vi "NOSAMSBouncerDAQrestartFC.vi"(8 "error in (no error)":errorcluster) -> (0 "error out":errorcluster, 2 "Summary Data":T3={"C12LE"=1.472651644671806e-07, "C13LE"=7.43208703350402e-08, "C12"=7.325707563373238e-08, "C13L"=240.0, "C13H"=6.302996266666667, "C1312"=6.305409493333333, "Counts"=0, "LT"=1.0021241544060013, "RT"=0.0, "BadBlocks"=0}, 3 "Run Average Ratios":T7={"C14Rate"=38.07712869341802, "CountErr"=0.06454972243679029, "DT"=0.002413226666666546, "DTfrac"=0.0003827232266545153, "C13"=307109705561.01575, "C13H/L"=0.9856864606602128, "d13C"=-48.24793286826845, "C14/13"=1.23985429323571e-10, "C12Cor"=28715190239906.207, "C13/12"=0.010695028328772694, "C14/12"=1.3260273874313845e-12, "LEC13/12"=0.0} {"LEC13/12" format="%_4e"; "DTfrac" format="%#_3g"; "DT" format="%#_3g"; "CountErr" format="%#_3g"; "d13C" format="%_4g"; "C13/12" format="%_4e"; "C14/12" format="%_4e"; "C14/13" format="%_3e"; "C12Cor" format="%_3e"; "C13" format="%_3e"; "C13H/L" format="%#_3g"})   [LabVIEW 2013]
uses:
  PixieKeithleyDAQstates.ctl
  <vilib>/DAQmx/configure/timing.llb/DAQmx Timing (Sample Clock).vi
  <vilib>/DAQmx/create/channels.llb/DAQmx Create Channel (AI-Voltage-Basic).vi
  <vilib>/DAQmx/create/channels.llb/DAQmx Create Channel (CI-Count Edges).vi
  <vilib>/DAQmx/read.llb/DAQmx Read (Counter U32 1Chan 1Samp).vi
  <vilib>/DAQmx/create/channels.llb/DAQmx Create Channel (CO-Pulse Generation-Time).vi
  <vilib>/DAQmx/configure/timing.llb/DAQmx Timing (Implicit).vi
  <vilib>/DAQmx/create/channels.llb/DAQmx Create Channel (AO-Voltage-Basic).vi
  <vilib>/DAQmx/configure/timing.llb/DAQmx Timing (Use Waveform).vi
  <vilib>/DAQmx/write.llb/DAQmx Write (Analog Wfm 1Chan NSamp).vi
  <resource>/objmgr/daqmx.rc
  <vilib>/DAQmx/configure/trigger.llb/DAQmx Start Trigger (Digital Edge).vi
  <vilib>/DAQmx/read.llb/DAQmx Read (Analog 1D Wfm NChan NSamp).vi
  RunRatios.ctl
  FCOffset.ctl
  SummaryData.ctl
  BouncerParameters.ctl
panel:
  out "Bouncer Waveform":waveform(dbl)(graph)
  in  "Bouncer Parameters":T1={"12C Period"=1.0, "12C Delay"=0.0, "12C Voltage"=9.022, "13C Period"=10.0, "13C Delay"=0.0, "13C Voltage"=5.239, "14C Period"=100.0, "14C Delay"=0.0, "14C Voltage"=2.0, "LE13C Period"=0.0, "LE13C Delay"=0.0, "LE13C Voltage"=0.0, "LE12C Period"=0.0, "LE12C Delay"=0.0, "LE12C Voltage"=0.0} {"LE12C Voltage" format="%_4f"; "LE13C Voltage" format="%_4f"}
  in  "samples per channel":i32=1000
  out "CH1 GDT":dbl
  out "CH0 GDT":dbl
  in  "FC Offset":T2={"HE 12C Offset"=0.0, "HE 13CL Offset"=0.0, "HE 13CH Offset"=0.0, "LE FC Scale"=0, "HE C12 Scale"=0, "HE C13 Scale"=18} {"HE C13 Scale" items=["500 mA/V", "200 mA/V", "100 mA/V", "50 mA/V", "20 mA/V", "10 mA/V", "5 mA/V", "2 mA/V", "1 mA/V", "500 uA/V", "200 uA/V", "100 uA/V", "50 uA/V", "20 uA/V", "10 uA/V", "5 uA/V", "2 uA/V", "1 uA/V", "500 nA/V", "200 nA/V", "100 nA/V", "50 nA/V", "20 nA/V", "10 nA/V", "5 nA/V", "2 nA/V", "1 nA/V", "500 pA/V", "200 pA/V", "100 pA/V", "50 pA/V", "20 pA/V", "10 pA/V", "5 pA/V", "2 pA/V", "1 pA/V", ""]; "HE C12 Scale" items=["500 mA/V", "200 mA/V", "100 mA/V", "50 mA/V", "20 mA/V", "10 mA/V", "5 mA/V", "2 mA/V", "1 mA/V", "500 uA/V", "200 uA/V", "100 uA/V", "50 uA/V", "20 uA/V", "10 uA/V", "5 uA/V", "2 uA/V", "1 uA/V", "500 nA/V", "200 nA/V", "100 nA/V", "50 nA/V", "20 nA/V", "10 nA/V", "5 nA/V", "2 nA/V", "1 nA/V", "500 pA/V", "200 pA/V", "100 pA/V", "50 pA/V", "20 pA/V", "10 pA/V", "5 pA/V", "2 pA/V", "1 pA/V", ""]; "LE FC Scale" items=["500 mA/V", "200 mA/V", "100 mA/V", "50 mA/V", "20 mA/V", "10 mA/V", "5 mA/V", "2 mA/V", "1 mA/V", "500 uA/V", "200 uA/V", "100 uA/V", "50 uA/V", "20 uA/V", "10 uA/V", "5 uA/V", "2 uA/V", "1 uA/V", "500 nA/V", "200 nA/V", "100 nA/V", "50 nA/V", "20 nA/V", "10 nA/V", "5 nA/V", "2 nA/V", "1 nA/V", "500 pA/V", "200 pA/V", "100 pA/V", "50 pA/V", "20 pA/V", "10 pA/V", "5 pA/V", "2 pA/V", "1 pA/V", ""]}
  out "HE 13CL Cup":waveform(dbl)(graph)={"t0"=timestamp(3415120333.4017754 s since 1904-01-01), "dt"=9.999999999999972e-06, "Y"=[0.41889009921070675, 0.6410939957678486, 0.7270772818431984, 0.7261111773784867, 0.7270772818431984, 0.7293315256055366, 0.7267552470213039, 0.7286874559575331, 0.7306196649054364, 0.7254671077369653, 0.7283654211340178, 0.7302976300799747, 0.7277213514879598, 0.7261111773784867, 0.7306196649054364, 0.7341620480069433, 0.7293315256055366, 0.7302976300799747, 0.7319078042105287, 0.7331959435208164, 0.7280433863108267, 0.7331959435208164, 0.7290094907813727, 0.7299755952548376, 0.7309416997312226, 0.7344840828363023, 0.7293315256055366, 0.7299755952548376, 0.7267552470213039, 0.7338400131779094, 0.7219247247317432, 0.7225687943661443, 0.7280433863108267, 0.7280433863108267, 0.7309416997312226, 0.7290094907813727, 0.7328739086927573, 0.7277213514879598, 0.7161280980802982, 0.7286874559575331], "attributes"=variant("NI_ChannelName"=variant(string "PXI1Slot2/ai2"), "NI_UnitDescription"=variant(string "Volts"))}
  out "Bouncer":waveform(dbl)(graph)={"t0"=timestamp(3415120333.4009705 s since 1904-01-01), "dt"=9.999999999999972e-06, "Y"=array[1000 elements], "attributes"=variant("NI_ChannelName"=variant(string "PXI1Slot2/ai0"), "NI_UnitDescription"=variant(string "Volts"))}
  out "LE 13C Cup":waveform(dbl)(graph)={"t0"=timestamp(3415120333.402178 s since 1904-01-01), "dt"=9.999999999999972e-06, "Y"=[0.8050097183722652, 0.24660166407635983, 0.028584441505206795, 0.009584422869030943, 0.009906457076575987, 0.00797425183471986, 0.00797425183471986, 0.007008149216862962, 0.012804764954733521, 0.01312679916455761, 0.010550525492349248, 0.010872559700577551, 0.009584422869030943, 0.01022849128434874, 0.01151662811771772, 0.010872559700577551, 0.010872559700577551, 0.010872559700577551, 0.01022849128434874, 0.009262388661713566, 0.004109841375562904, 0.009262388661713566, 0.01151662811771772, 0.01022849128434874, 0.019567483409006912, 0.01151662811771772, 0.010872559700577551, 0.009906457076575987, 0.009584422869030943, 0.01022849128434874, 0.013448833374609843, 0.01022849128434874, 0.009906457076575987, 0.010550525492349248, 0.00668611501136536, 0.010550525492349248, 0.01022849128434874, 0.01022849128434874, 0.009584422869030943, 0.013448833374609843], "attributes"=variant("NI_ChannelName"=variant(string "PXI1Slot2/ai3"), "NI_UnitDescription"=variant(string "Volts"))}
  out "LE 12C Cup":waveform(dbl)(graph)={"t0"=timestamp(3415120333.4013777 s since 1904-01-01), "dt"=9.999999999999972e-06, "Y"=[0.00668611501136536, 0.007008149216862962, 0.007652217628540168, 0.007330183422587883, 0.00861832024776164, 0.007330183422587883, 0.009262388661713566, 0.01312679916455761, 0.05338107720327494, 0.6781279926088322, 0.8175690797952145, 0.8223996035554544, 0.8240097781590372, 0.8233657083165931, 0.8249758829252316, 0.8230436733958766, 0.8243318130807649, 0.8236877432376466, 0.8243318130807649, 0.8243318130807649, 0.8233657083165931, 0.8278741972420289, 0.8236877432376466, 0.8240097781590372, 0.8227216384754971, 0.8246538480028296, 0.8246538480028296, 0.8246538480028296, 0.8249758829252316, 0.8252979178479707, 0.8214334987973474, 0.8236877432376466, 0.8246538480028296, 0.8246538480028296, 0.8227216384754971, 0.8236877432376466, 0.8243318130807649, 0.8217555337163797, 0.8240097781590372, 0.8243318130807649], "attributes"=variant("NI_ChannelName"=variant(string "PXI1Slot2/ai3"), "NI_UnitDescription"=variant(string "Volts"))}
  out "HE 13CH Cup":waveform(dbl)(graph)={"t0"=timestamp(3415120333.4017754 s since 1904-01-01), "dt"=9.999999999999972e-06, "Y"=[0.41889009921070675, 0.6410939957678486, 0.7270772818431984, 0.7261111773784867, 0.7270772818431984, 0.7293315256055366, 0.7267552470213039, 0.7286874559575331, 0.7306196649054364, 0.7254671077369653, 0.7283654211340178, 0.7302976300799747, 0.7277213514879598, 0.7261111773784867, 0.7306196649054364, 0.7341620480069433, 0.7293315256055366, 0.7302976300799747, 0.7319078042105287, 0.7331959435208164, 0.7280433863108267, 0.7331959435208164, 0.7290094907813727, 0.7299755952548376, 0.7309416997312226, 0.7344840828363023, 0.7293315256055366, 0.7299755952548376, 0.7267552470213039, 0.7338400131779094, 0.7219247247317432, 0.7225687943661443, 0.7280433863108267, 0.7280433863108267, 0.7309416997312226, 0.7290094907813727, 0.7328739086927573, 0.7277213514879598, 0.7161280980802982, 0.7286874559575331], "attributes"=variant("NI_ChannelName"=variant(string "PXI1Slot2/ai2"), "NI_UnitDescription"=variant(string "Volts"))}
  out "HE 12C Cup":waveform(dbl)(graph)={"t0"=timestamp(3415120333.400973 s since 1904-01-01), "dt"=9.999999999999972e-06, "Y"=[-0.00168677425192447, 0.003143738765882537, -0.002652876849375083, -0.00168677425192447, 0.0008894993512310448, -0.002652876849375083, 0.0005674651500443148, -0.000720671652438485, 0.0018556019561503992, 0.0018556019561503992, 0.0024996703605630385, 0.0015335677542840436, 0.002177636158243383, -0.0013647400523220184, 0.005397978191647298, 0.0018556019561503992, 0.0012115335526442733, 0.0015335677542840436, 0.016669175487689536, 0.2607711773435167, 0.6375516136789285, 0.6369075442122739, 0.6423821347186465, 0.6456024821175347, 0.6449584126352536, 0.6423821347186465, 0.6456024821175347, 0.6427041694571275, 0.639805856822051, 0.6427041694571275, 0.6388397526159826, 0.6449584126352536, 0.6423821347186465, 0.6443143431542244, 0.6452804473762376, 0.6401278915580318, 0.6410939957678486, 0.6468906210858548, 0.6446363778945825, 0.6433482389350278], "attributes"=variant("NI_ChannelName"=variant(string "PXI1Slot2/ai1"), "NI_UnitDescription"=variant(string "Volts"))}
  out "C13LE":dbl=7.360825676338929e-08 format="%_4g"
  out "C12LE":dbl=7.360825676338929e-08 format="%_4g"
  in  "SampClk.Rate":dbl=10000.0
  out "DT Corrected Rate":dbl=38.103932081925684
  out "SCA Rate":dbl=38.473667612740456
  out "SCA Counts":u32=244
  out "CH1 SFDT":dbl=0.004433706666666666 format="%#_2f"
  out "CH0 SFDT":dbl=0.004324053333333333 format="%#_2f"
  in  "Mode":enum16{"Tuning", "Run", "Manual"}(ring)
  out "Block Spectrum":u32[][](graph) caption="ADC Spectrum"
  out "RunningAverages":T3={"C12LE"=1.4726514132603862e-07, "C13LE"=7.431122697335651e-08, "C12"=7.326197420828519e-08, "C13L"=222.0, "C13H"=5.887767893333334, "C1312"=5.884231466666667, "Counts"=0, "LT"=1.0020921000294485, "RT"=0.0, "BadBlocks"=0}
  out "Elapsed Time":dbl=6.3420000000000005
  out "element":T4=enum."Idle"
  in  "Stop":bool
  in  "Stop DAQ":bool
  in  "Run Parameters":T5={"Block time (s)"=0.2, "Max Runtime (s)"=100000.0, "Max Counts"=100000, "C12 Limit"=-1.0, "Max BadBlocks"=100} {"Block time (s)" min=0.0 max=100.0 step=0.1}
  out "Acquiring":bool
  in  "StartDAQ":bool
  in  "Logfile":string="Feb12.txt"
  in  "Log File Path":path=path "C:/DAQ Logs"
  out "Good Block":bool=TRUE
  out "Currents & Counts":cluster{dbl, dbl, dbl, dbl, dbl}(graph)
  out "Ratios":T6(graph)={"C14/12"=1.3260273874313845e-12, "C14/12"=1.3130784198635677e-12, "d13C"=-48.24793286826845, "d13C"=-48.27837602145524}
  out "13C H/L":dbl(knob)=0.9886607752123965 scale=0.0..2.0 scale format="%#_3g"
  out "Currents":cluster{dbl, dbl}(knob)={1.4754487124301994e-07, 1.4806074705013686e-07} scale=0.0..1e-06 scale format="%#_1e"
  out "12/13":dbl=93.50437948492602
  out "Ch1 Rate 2":cluster{dbl, "Ch1 Rate":dbl}(graph)={38.07712869341802, "Ch1 Rate"=37.7052907013146}
  out "Moving Averages":T7={"C14Rate"=37.7052907013146, "CountErr"=0.06711560552140243, "DT"=-0.0035364266666668698, "DTfrac"=-0.0006010006041910865, "C13"=307099831658.9964, "C13H/L"=0.9858802928197172, "d13C"=-48.27837602145524, "C14/13"=1.2277861077821284e-10, "C12Cor"=28715185727621.875, "C13/12"=0.010694686232971703, "C14/12"=1.3130784198635677e-12, "LEC13/12"=0.0} {"LEC13/12" format="%_4e"; "DTfrac" format="%#_3g"; "DT" format="%#_3g"; "CountErr" format="%#_3g"; "d13C" format="%_4g"; "C13/12" format="%_4e"; "C14/12" format="%_4e"; "C14/13" format="%_3e"; "C12Cor" format="%_3e"; "C13" format="%_3e"; "C13H/L" format="%#_3g"}
  in  "CountPoints":i32=30 min=1
  in  "CurPoints":i32=30 min=1
  out "C12":dbl=1.4754487124301994e-07 format="%_4g"
  out "C13L":dbl=7.445249028674759e-08 format="%_4g"
  out "C13H":dbl=7.360825676338929e-08 format="%_4g"
  out "Run time [s]":dbl=6.305409493333333 format="%_6g"
  out "Ch1 LT":dbl=6.302996266666667
  out "Ch1 Counts":u32=240
  out "Ch1 Rate":dbl=38.07712869341802
  out "Ch0 LT":dbl=6.305354879999999
  out "Ch0 Counts":u32=243
  out "Ch0 Rate":dbl=38.53867143477895
  # "Currents"
  # "Counts"
  # "Livetime"
  # "Rate"
  # "SFDT"
  # "GDT"
  # "Cor Rate"
  # "Ch 0"
  # "Ch1"
  # "SCA"
  # "ms"
  # "us"
  # "kV"
  # "ms"
  # "us"
  # "kV"
  # "ms"
  # "us"
  # "kV"
  # "ms"
  # "us"
  # "kV"
  # "ms"
  # "us"
  # "kV"
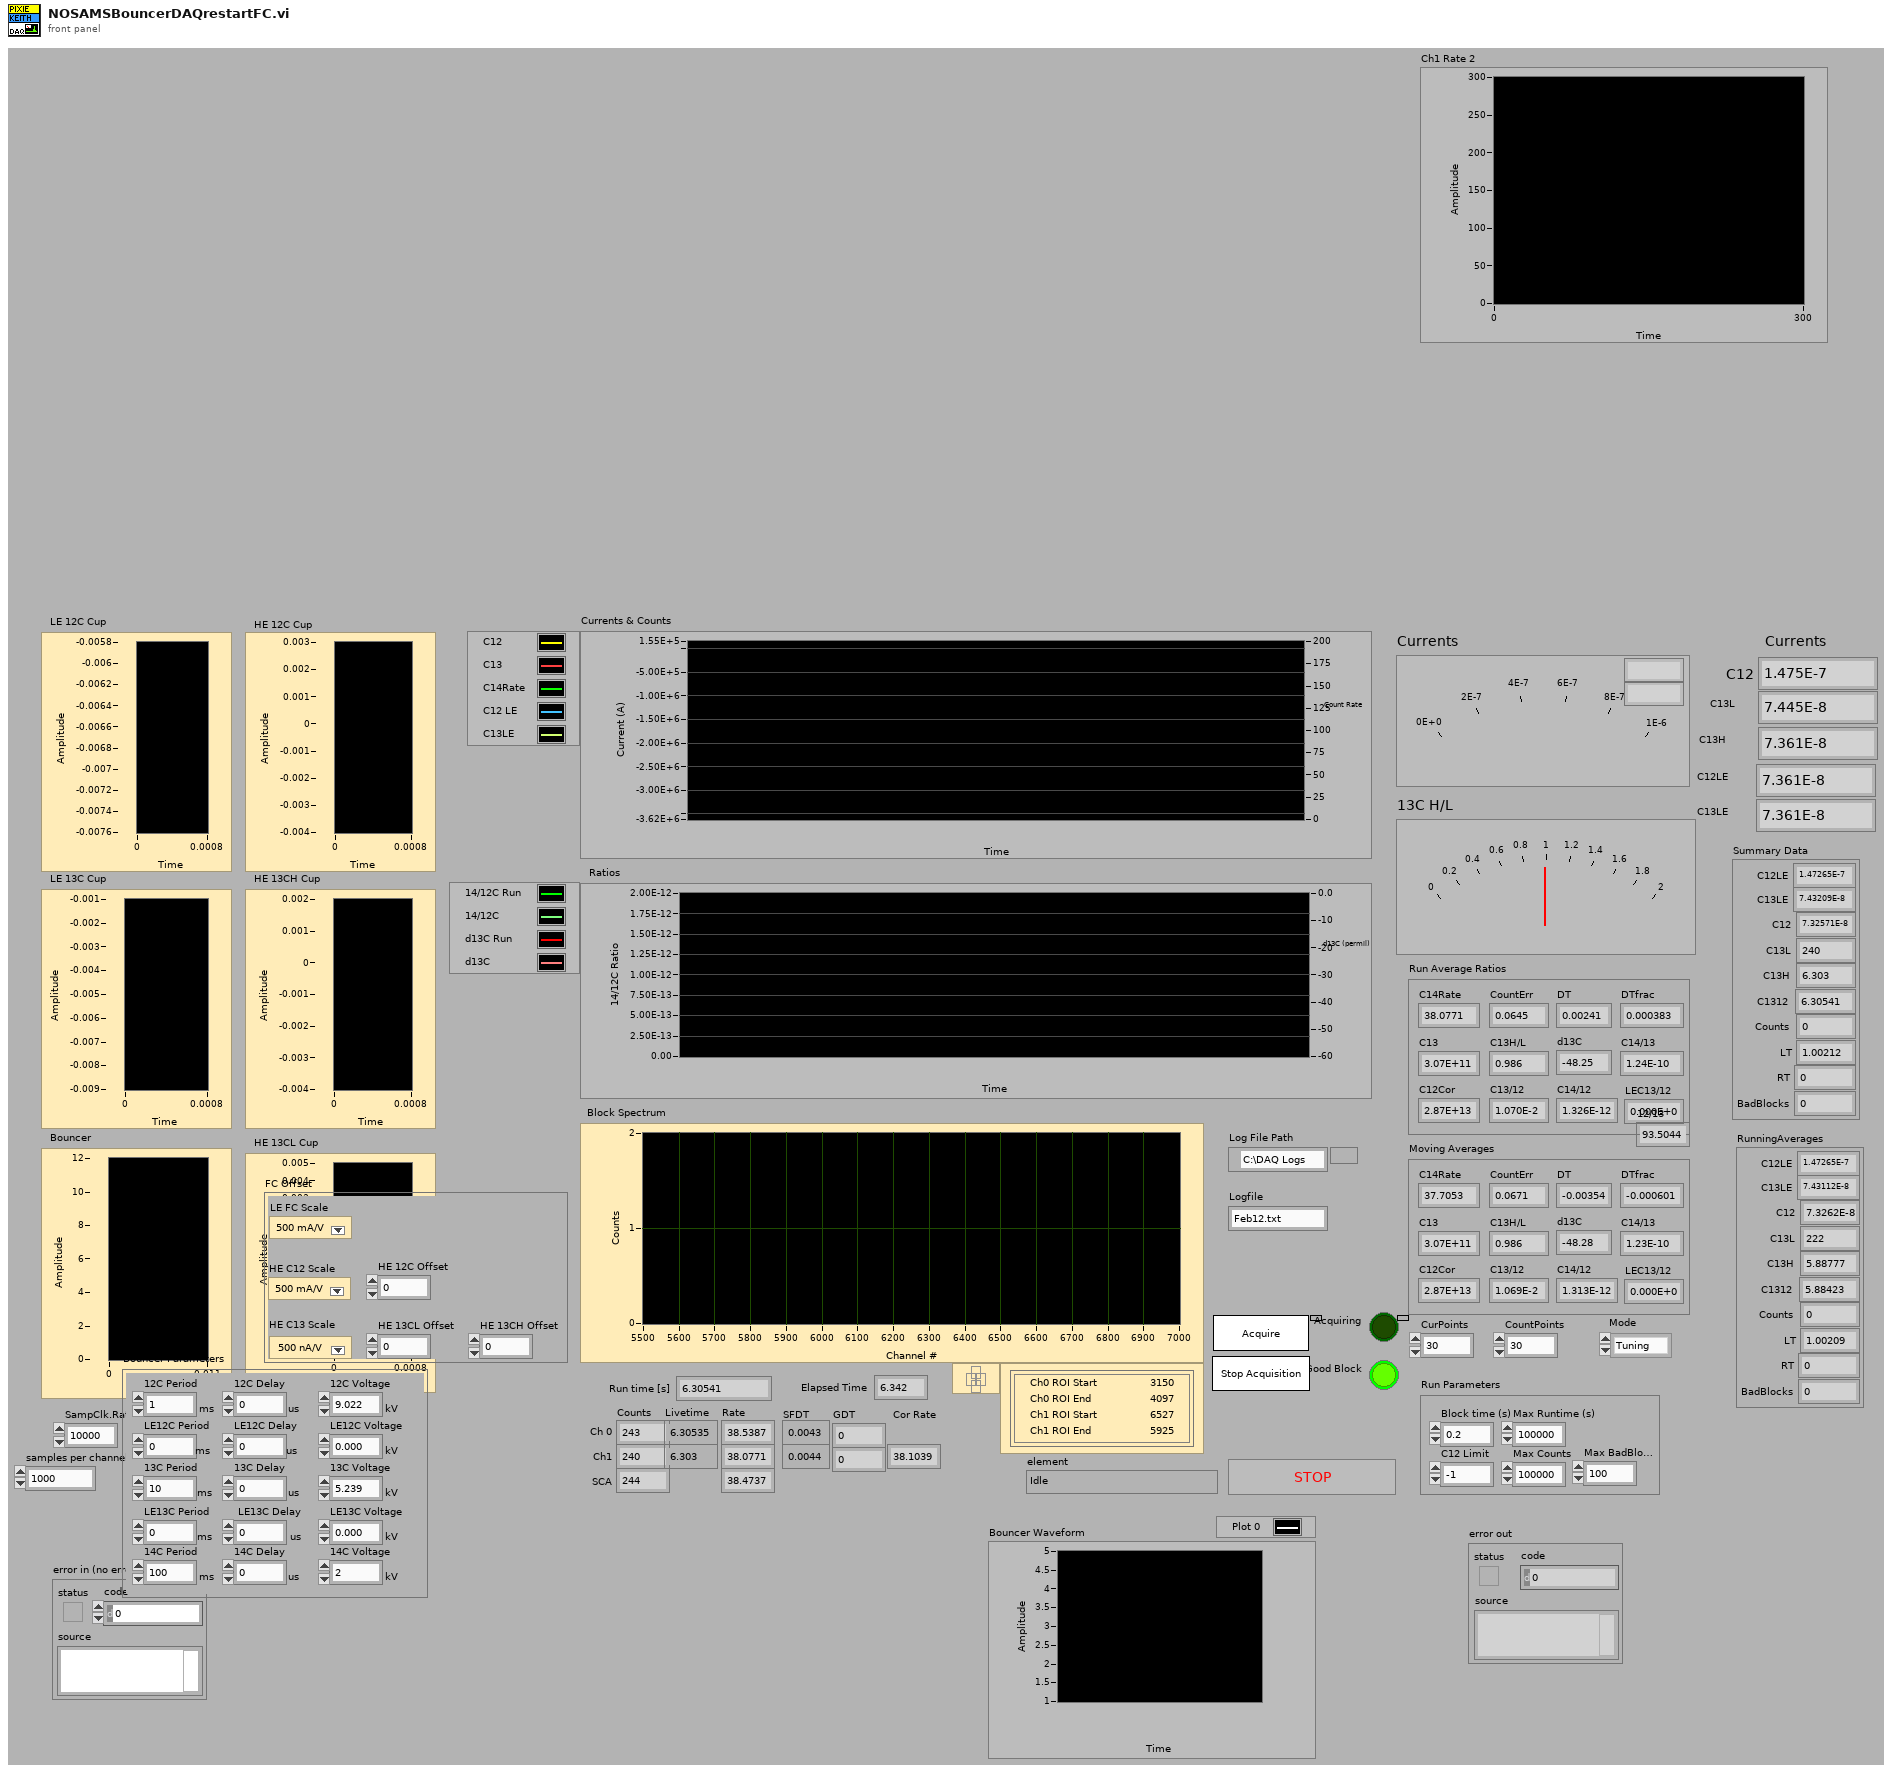
[diagram p1: front panel]
types:
  T1 = typedef "BouncerParameters.ctl" = cluster{"12C Period":dbl, "12C Delay":dbl, "12C Voltage":dbl, "13C Period":dbl, "13C Delay":dbl, "13C Voltage":dbl, "14C Period":dbl, "14C Delay":dbl, "14C Voltage":dbl, "LE13C Period":dbl, "LE13C Delay":dbl, "LE13C Voltage":dbl, "LE12C Period":dbl, "LE12C Delay":dbl, "LE12C Voltage":dbl}
  T2 = typedef "FCOffset.ctl" = cluster{"HE 12C Offset":dbl, "HE 13CL Offset":dbl, "HE 13CH Offset":dbl, "LE FC Scale":u16, "HE C12 Scale":u16, "HE C13 Scale":u16}
  T3 = typedef "SummaryData.ctl" = cluster{"C12LE":dbl, "C13LE":dbl, "C12":dbl, "C13L":dbl, "C13H":dbl, "C1312":dbl, "Counts":u32, "LT":dbl, "RT":dbl, "BadBlocks":u8}
  T4 = typedef "PixieKeithleyDAQstates.ctl" = enum16{"Initialize", "Restart Bouncer", "Idle", "Load Wheel", "Load Sample", "Start Run", "Wait", "Get Block", "Check Data", "Check Run", "Check Sample", "Analyse and Display", "Stop DAQ", "Log Data", "Stop"}
  T5 = cluster{"Block time (s)":dbl, "Max Runtime (s)":dbl, "Max Counts":u32, "C12 Limit":dbl, "Max BadBlocks":u8}
  T6 = cluster{"C14/12":dbl, "C14/12":dbl, "d13C":dbl, "d13C":dbl}
  T7 = typedef "RunRatios.ctl" = cluster{"C14Rate":dbl, "CountErr":dbl, "DT":dbl, "DTfrac":dbl, "C13":dbl, "C13H/L":dbl, "d13C":dbl, "C14/13":dbl, "C12Cor":dbl, "C13/12":dbl, "C14/12":dbl, "LEC13/12":dbl}
  T8 = typedef "BlockData.ctl" = cluster{"LE C12":dbl[], "LE C13":dbl[], "C12":dbl[], "C13L":dbl[], "C13H":dbl[], "C1312":dbl[], "Counts":u32[], "LT":dbl[], "RT":dbl[]}
  T9 = typedef "PixieTimes.ctl" = cluster{"CH0 LT":dbl, "CH1 LT":dbl, "CH0 SFDT":dbl, "CH1 SFDT":dbl, "CH0 GDT":dbl, "CH1 GDT":dbl, "Run time [s]":dbl}
  T10 = typedef "LVCursorListTypeDef.ctl" = cluster{"Name":string, "Color":u32, "Style":u8, "Point Style":u8, "Name Visible":bool, "Allow Drag":bool, "Cursor Mode":u32, "Plot":i32, "Index":i32, "Position":cluster{"X":dbl, "Y":dbl}, "X Scale":u32, "Y Scale":u32, "Watch Plots":i32[], "Watch All Plots":bool, "Plot Area":i32, "Label Offset":cluster{"X":dbl, "Y":dbl}}[]
  T11 = cluster{"Ch0 Counts":u32, "Ch0 Rate":dbl, "Ch1 Counts":u32, "Ch1 Rate":dbl}
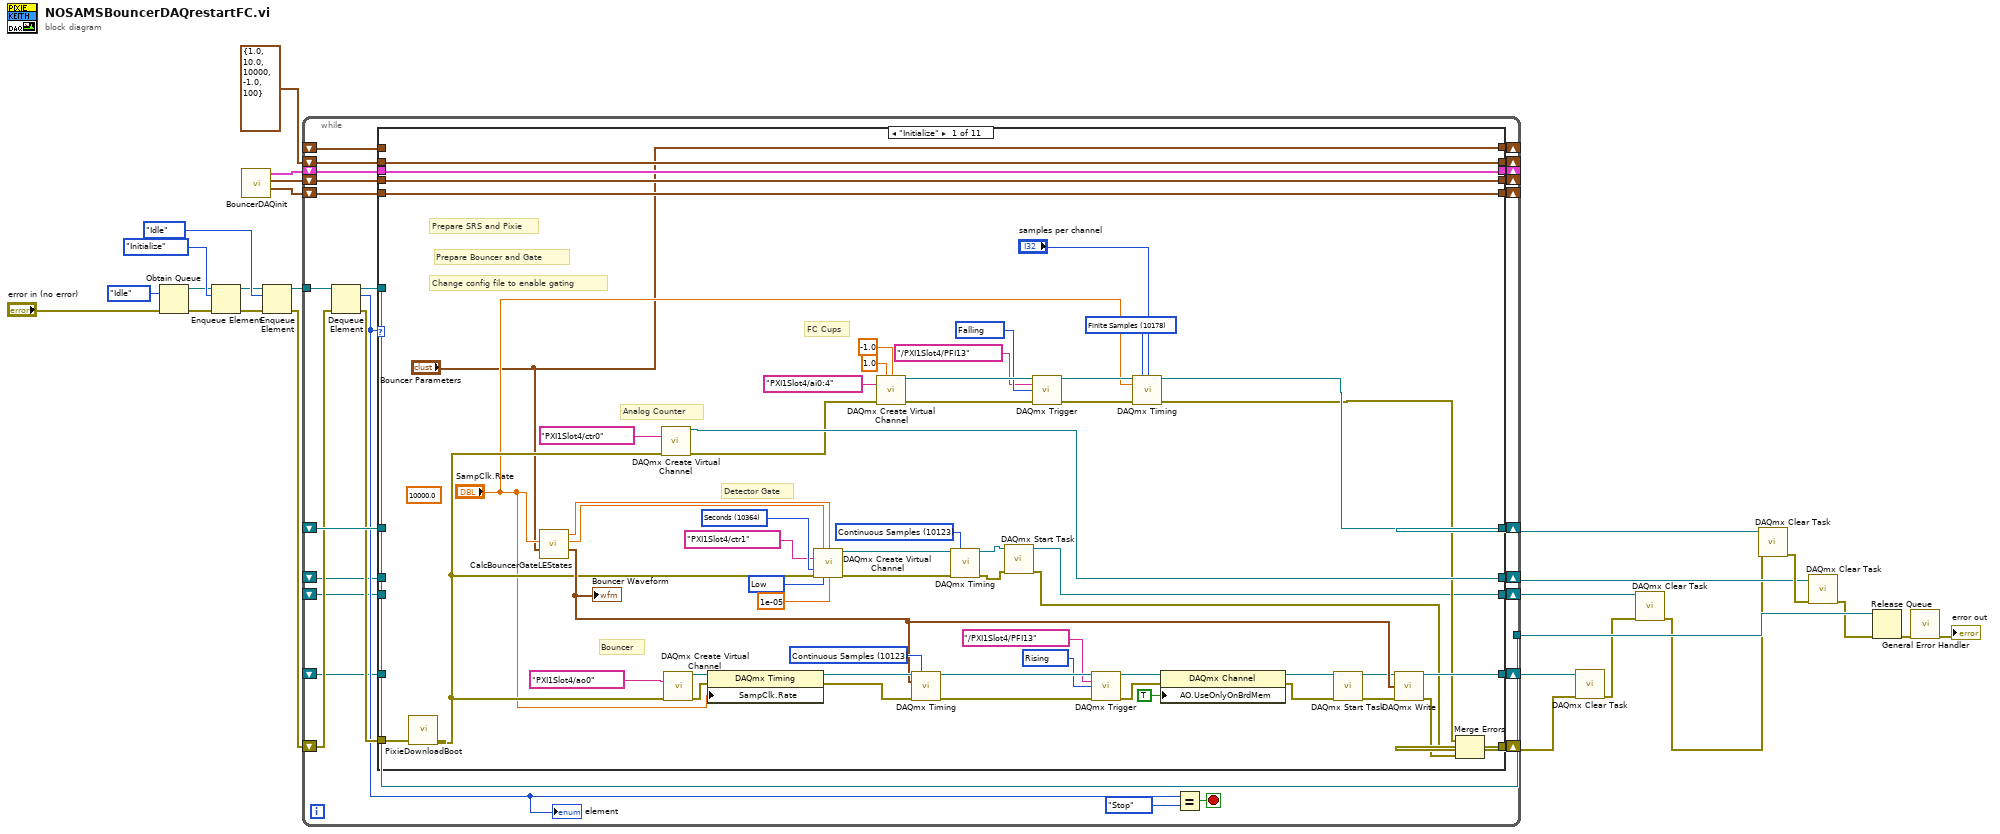
[diagram p0: block diagram]
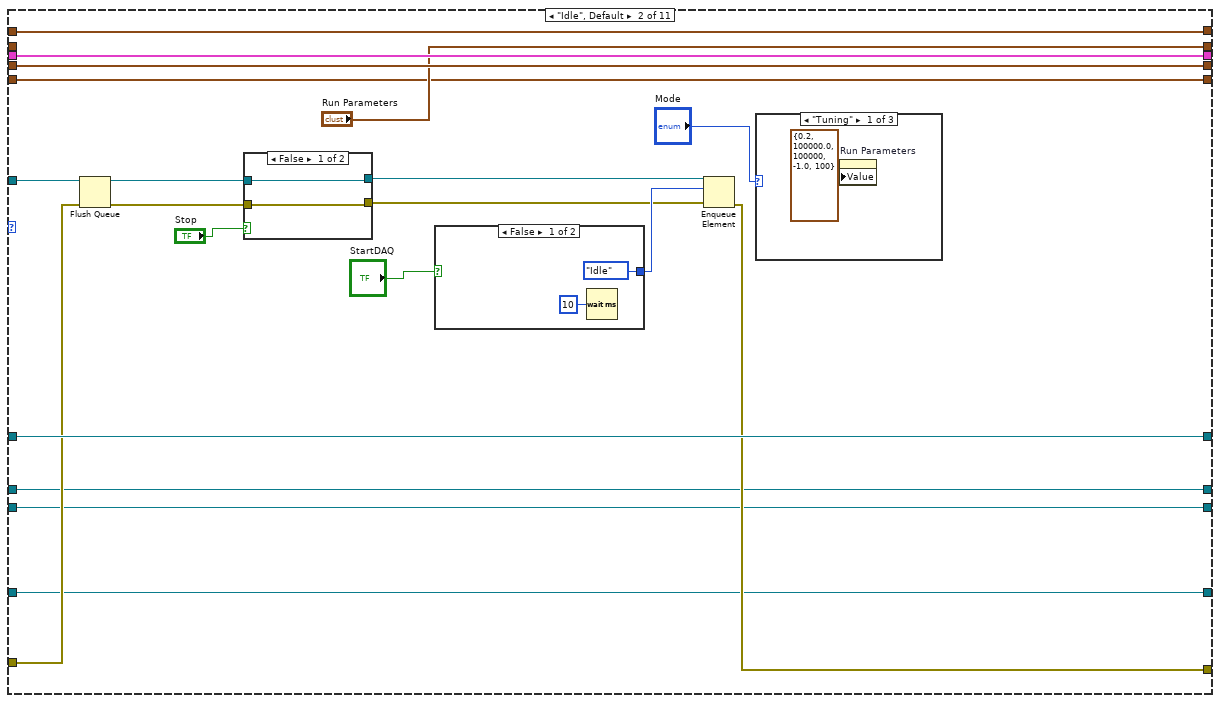
[diagram p2: hidden frame]
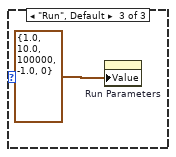
[diagram p4: hidden frame]
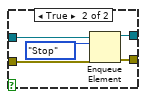
[diagram p5: hidden frame]
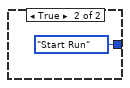
[diagram p6: hidden frame]
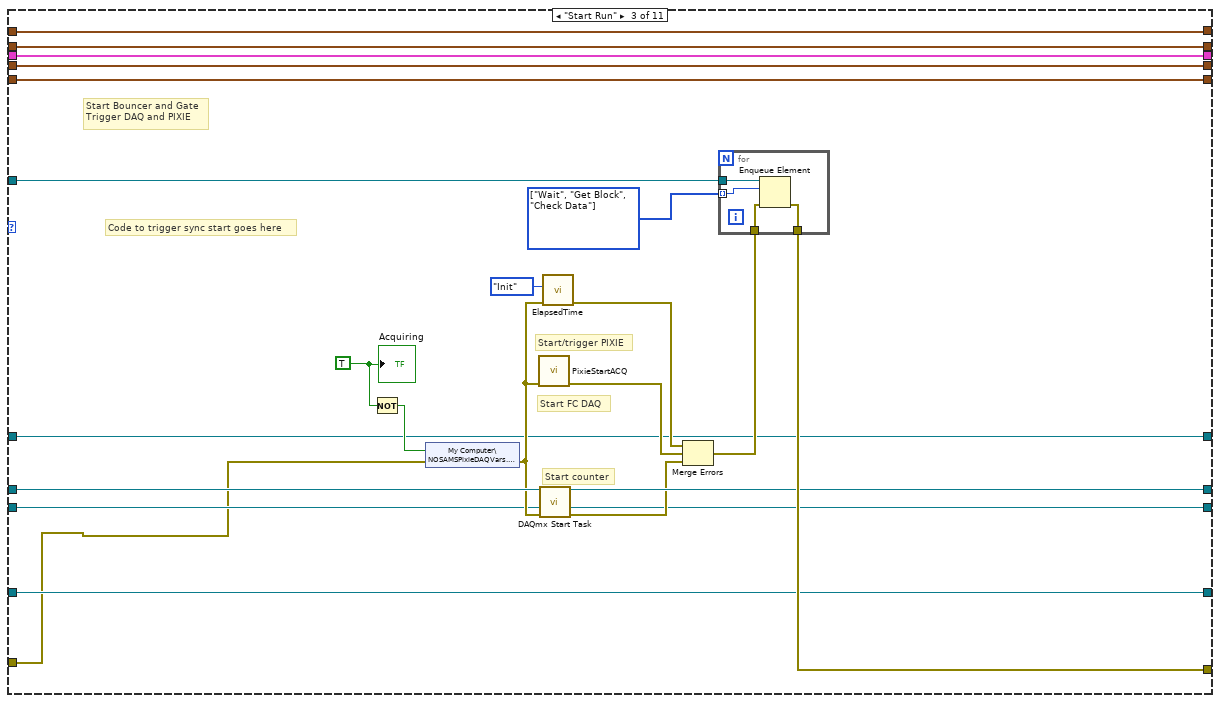
[diagram p7: hidden frame]
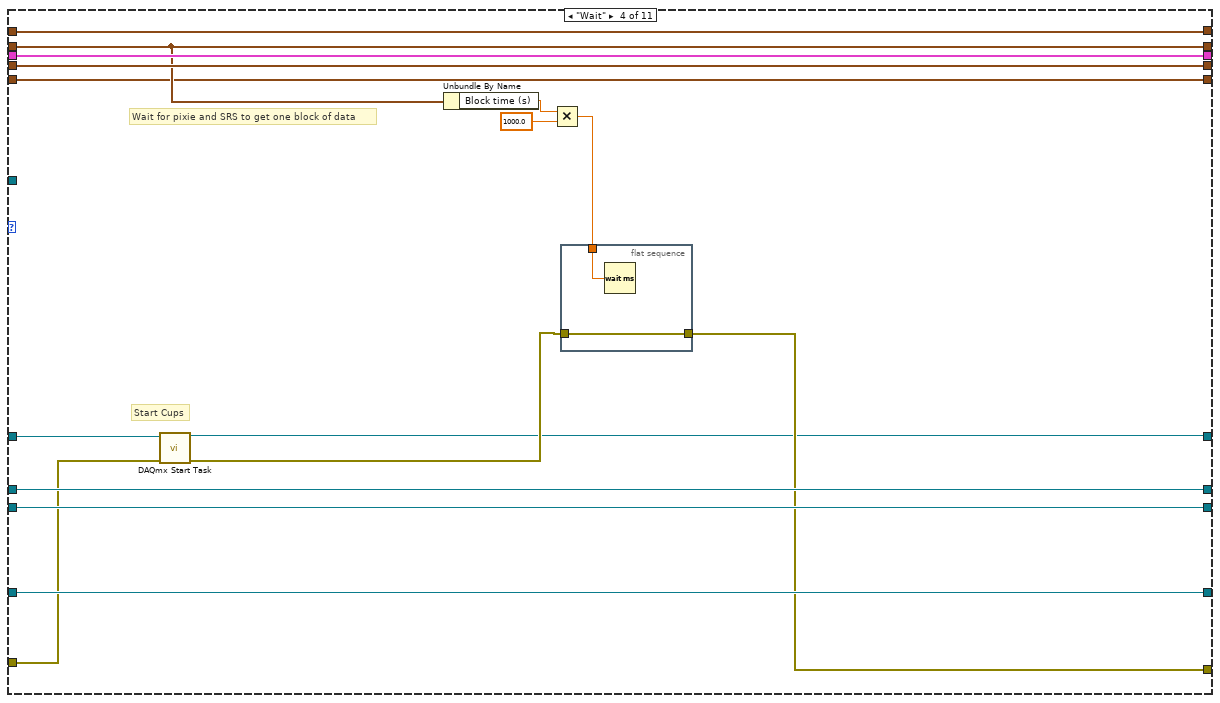
[diagram p8: hidden frame]
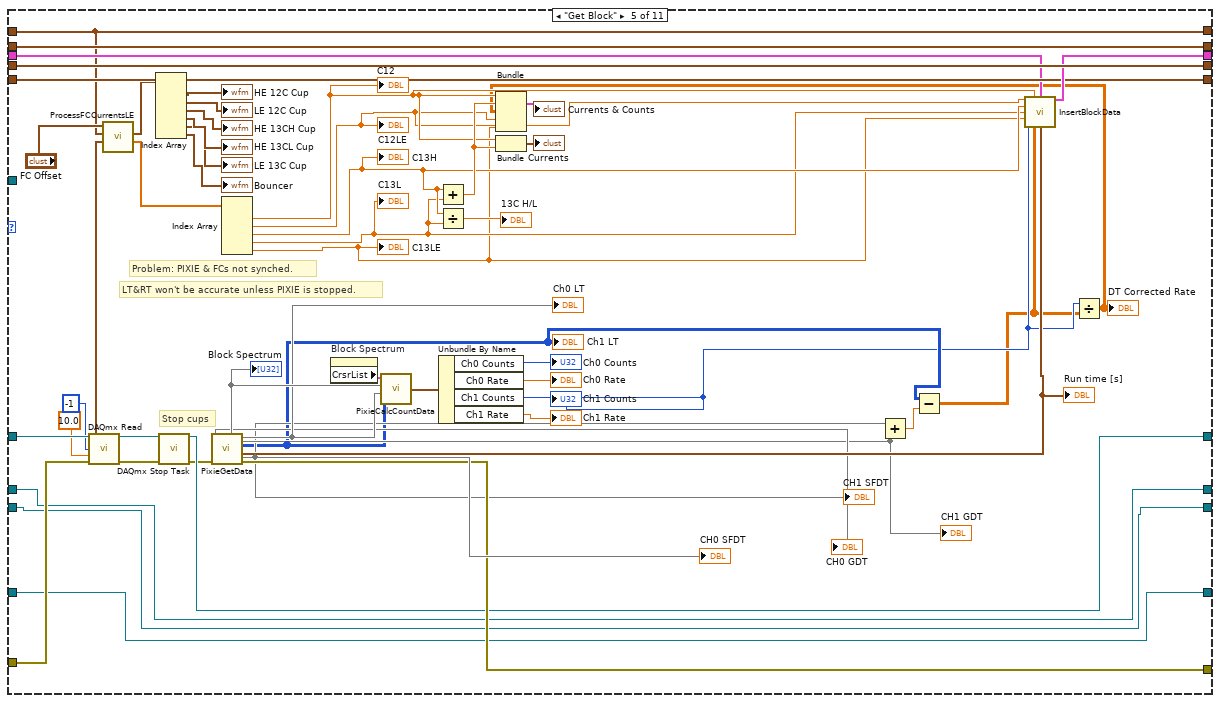
[diagram p9: hidden frame]
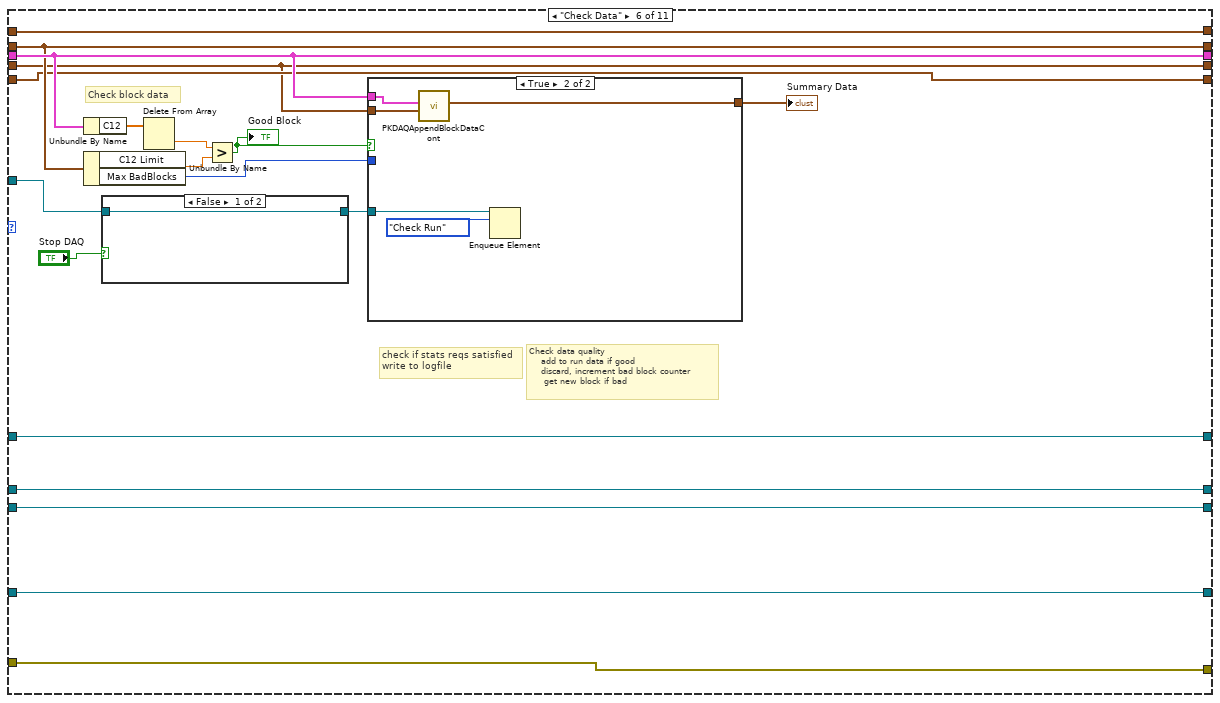
[diagram p10: hidden frame]
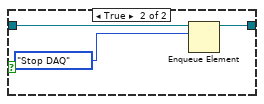
[diagram p11: hidden frame]
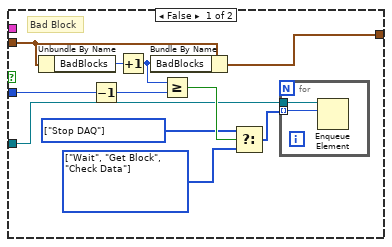
[diagram p12: hidden frame]
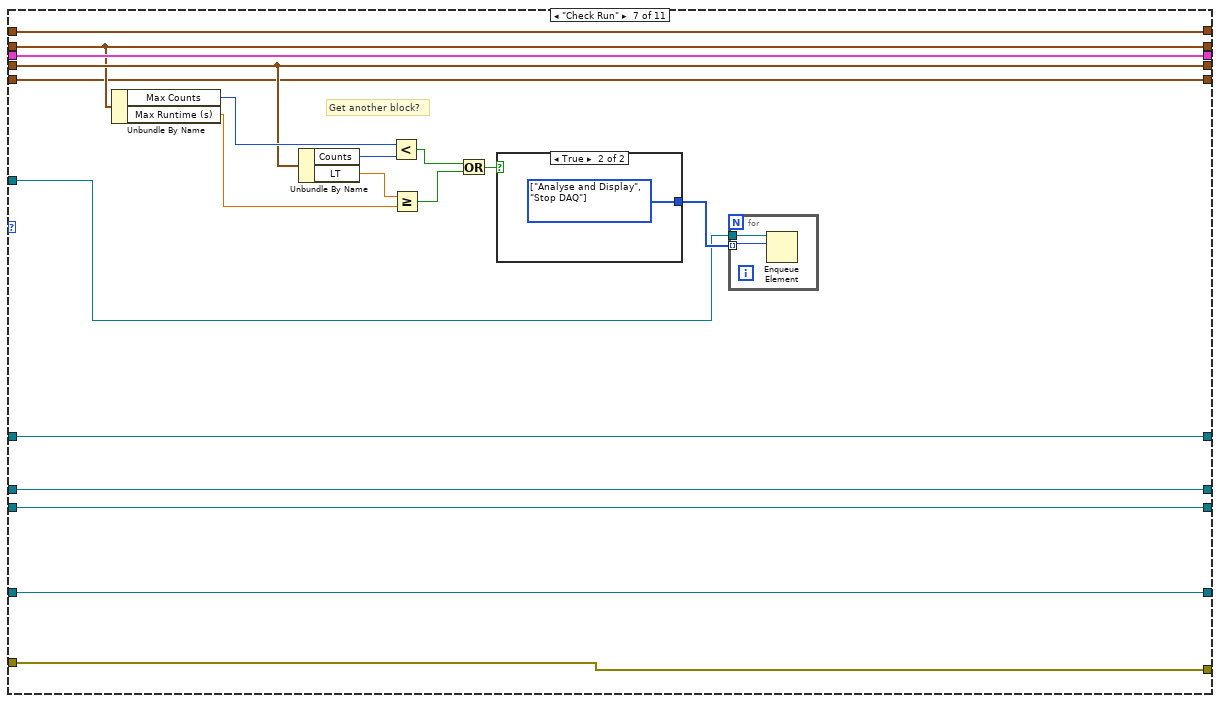
[diagram p13: hidden frame]
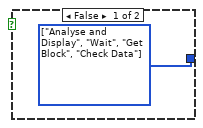
[diagram p14: hidden frame]
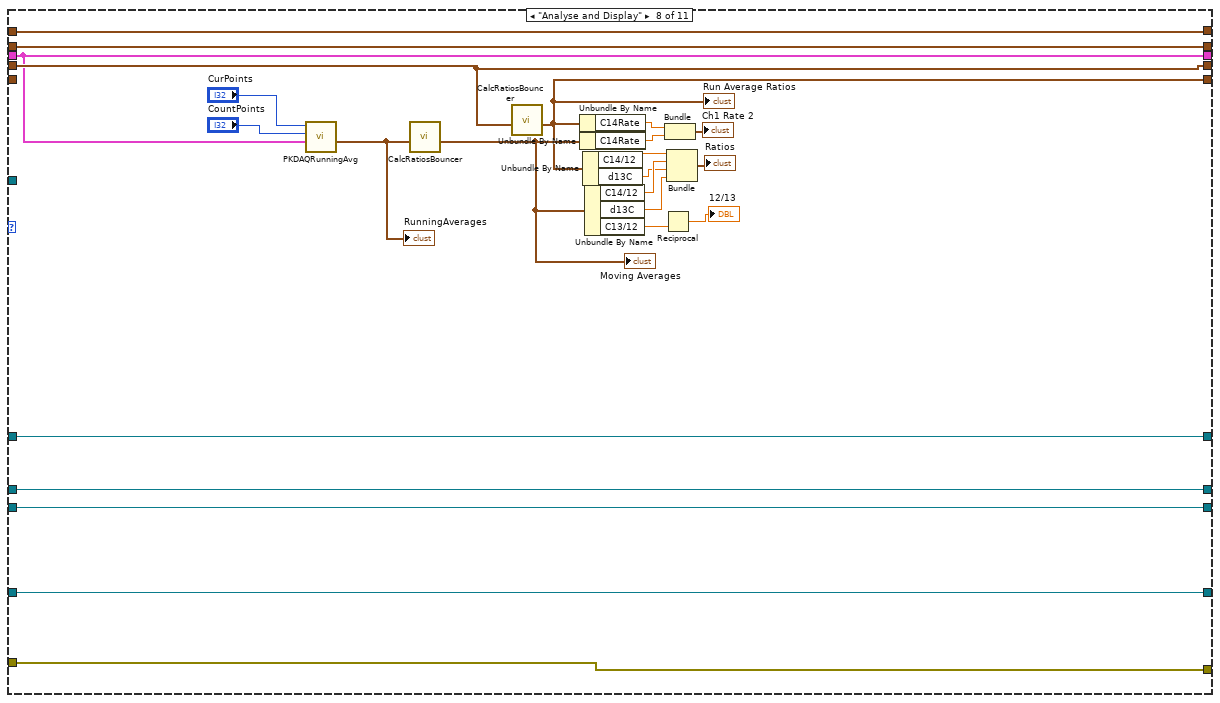
[diagram p15: hidden frame]
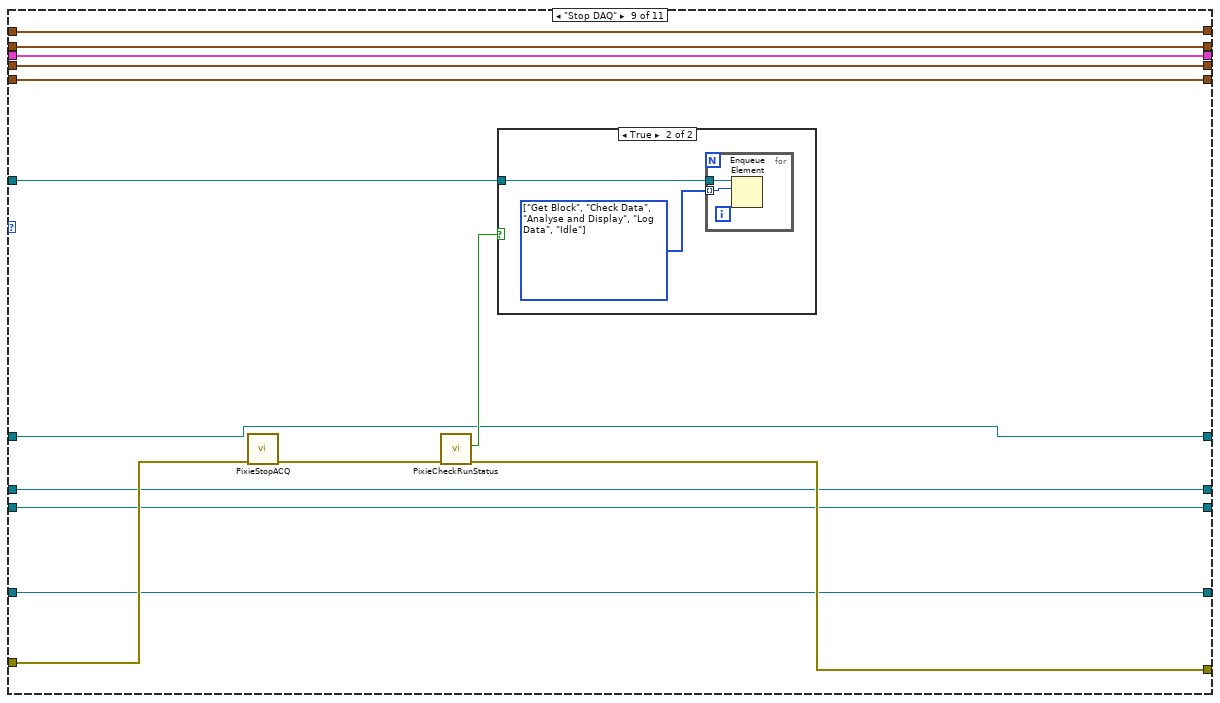
[diagram p16: hidden frame]
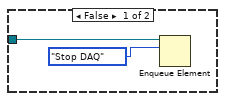
[diagram p17: hidden frame]
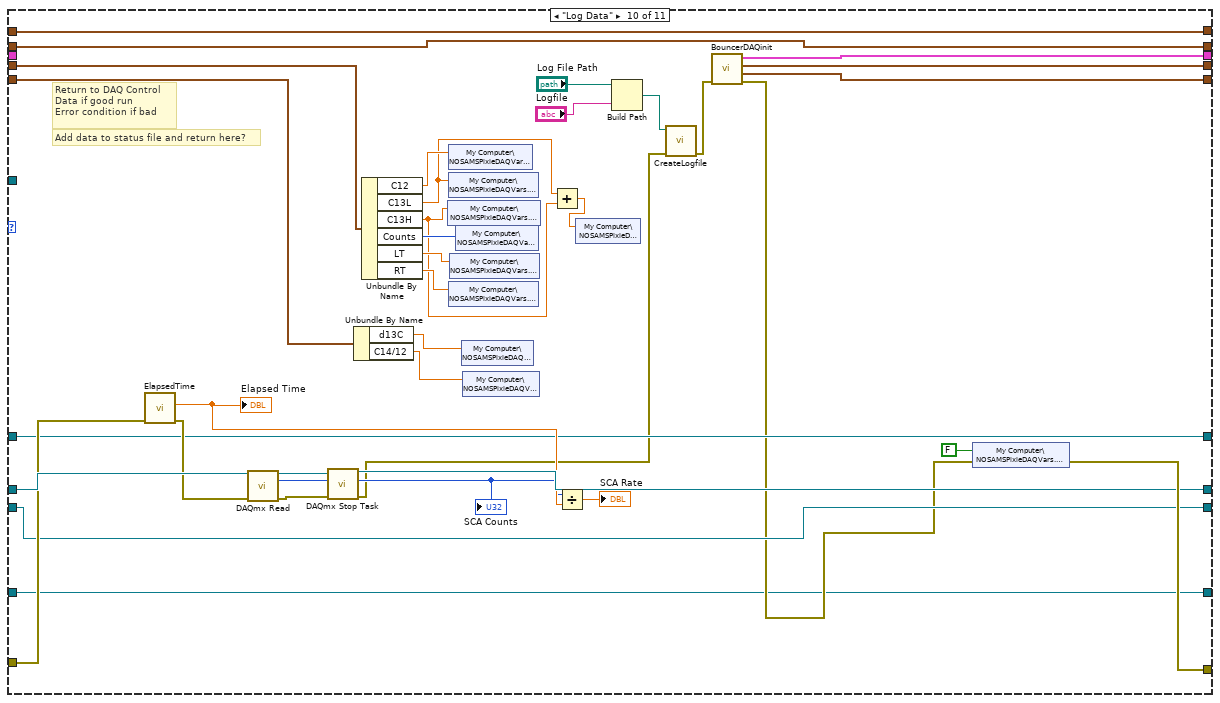
[diagram p18: hidden frame]
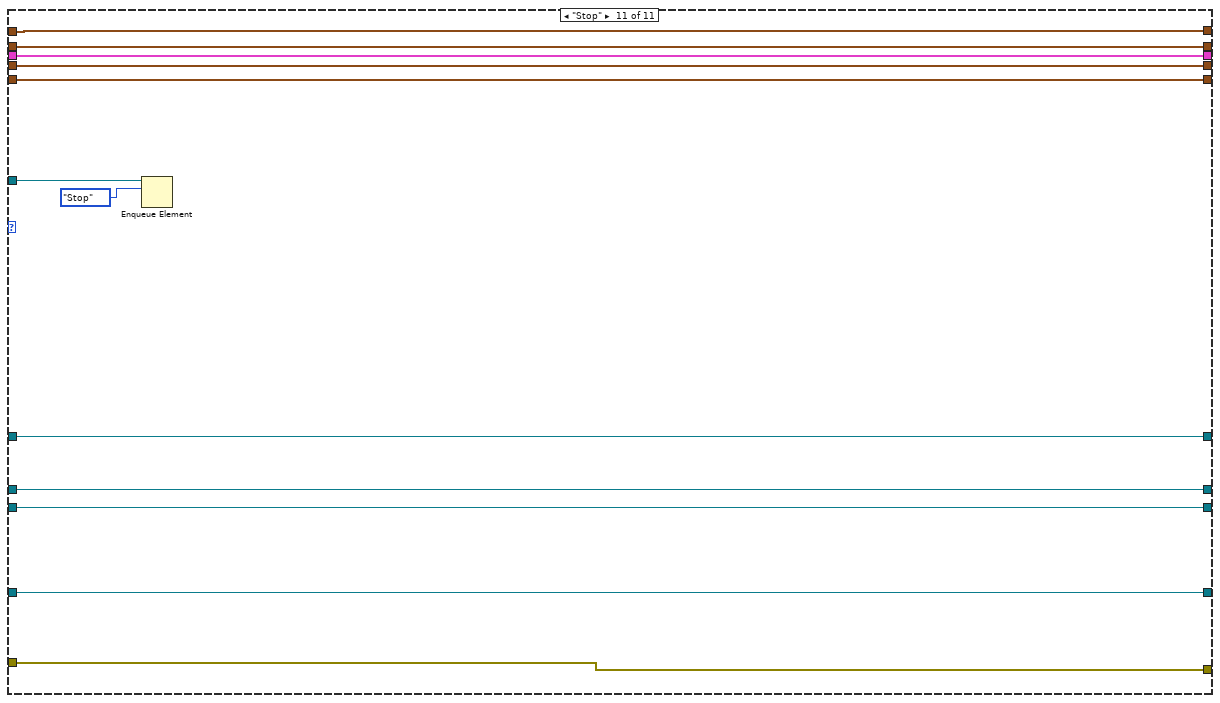
[diagram p19: hidden frame]
diagram:
  n1 = Obtain Queue(element data type=PixieKeithleyDAQstates."Idle" ("Next State"), error in (no error)="error in (no error)") -> (queue out=w16:refnum<queue>, error out=w15:errorcluster)  [unwired: 2 in, 2 out]
  n2 = Enqueue Element(queue=w16, element=PixieKeithleyDAQstates."Initialize", error in (no error)=w15) -> (queue out=w18:refnum<queue>, error out=w17:errorcluster)  [unwired: 2 out]
  n3 = call "BouncerDAQinit.vi"() -> ("Run Ratios"=w11:T7, "Summary Data"=w10:T3, "Block Data"=w9:T8)  [unwired: 2 in, 7 out]
  n4 = Enqueue Element(queue=w18, element=PixieKeithleyDAQstates."Idle", error in (no error)=w17) -> (queue out=w23:refnum<queue>, error out=w22:errorcluster)  [unwired: 2 out]
  n5 = while {
    shift-right: [w48] -> _
    shift-left: w9 -> [w49]
    shift-right: [w46] -> _
    shift-left: w10 -> [w47]
    shift-right: [w45] -> w26
    shift-left: _ -> [w44]
    shift-right: [w50] -> w2
    shift-left: w22 -> [w41]
    tunnel: w23 -> [w43]
    tunnel: [w40] -> w20
    shift-right: [w39] -> _
    shift-left: T5 {"Block time (s)"=1.0, "Max Runtime (s)"=10.0, "Max Counts"=10000, "C12 Limit"=-1.0, "Max BadBlocks"=100} ("Run Parameters 2") -> [w38]
    shift-right: [w35] -> _
    shift-left: w11 -> [w36]
    shift-right: [w34] -> w6
    shift-left: _ -> [w33]
    shift-right: [w32] -> w4
    shift-left: _ -> [w29]
    shift-right: [w31] -> w5
    shift-left: _ -> [w30]
    shift-right: [w28] -> _
    shift-left: _ -> [w27]
    stop <- w52 stop-if-true
    n6 = Dequeue Element(queue=w43, error in (no error)=w41) -> (queue out=w40:refnum<queue>, element=w37:T4, error out=w42:errorcluster)  [unwired: 2 out]
    "element" <- w37
    n7 = case shown="\"Initialize\"" w37 {
      tunnel: [w67 w122 w155 w172 w214 w259 w300 w328 w334 w377 w391] -> w50
      tunnel: w42 -> [w104 w124 w144 w173 w215 w259 w300 w328 w336 w360 w391]
      tunnel: w49 -> [w110 w130 w164 w184 w216 w253 w296 w306 w342 _ w396]
      tunnel: [w110 w130 w164 w184 w235 w253 w296 w306 w342 w371 w396] -> w48
      tunnel: w47 -> [w109 w129 w163 w183 w236 w242 w293 w307 w341 w355 w395]
      tunnel: [w109 w129 w163 w183 w236 w242 w293 w307 w341 w372 w395] -> w46
      tunnel: w38 -> [w103 _ w154 w179 w228 w249 w289 w312 w335 w379 w390]
      tunnel: [w64 w128 w147 w170 w190 w257 w297 w327 w337 w354 w392] -> w45
      tunnel: w44 -> [_ w128 w147 w171 w240 w257 w297 w327 w337 w354 w392]
      tunnel: w40 -> [_ w127 w159 _ _ w251 w287 _ w338 _ w393]
      tunnel: [w103 "Run Parameters" w154 w179 w228 w249 w289 w312 w335 w379 w390] -> w39
      tunnel: w36 -> [w102 w115 w152 w178 w226 w247 w286 _ w333 w370 w389]
      tunnel: [w102 w115 w152 w178 w226 w247 w286 w311 w333 w373 w389] -> w35
      tunnel: [w100 w114 w150 w177 w213 w246 w285 w310 w332 w361 w388] -> w34
      tunnel: w33 -> [_ w114 w151 w177 w213 w246 w285 w310 w332 w364 w388]
      tunnel: [w76 w112 w146 w175 w211 w244 w283 w308 w330 w350 w386] -> w32
      tunnel: [w56 w113 w145 w176 w212 w245 w284 w309 w331 w352 w387] -> w31
      tunnel: w30 -> [_ w113 w145 w176 w212 w245 w284 w309 w331 w352 w387]
      tunnel: w29 -> [_ w112 w146 w175 w211 w244 w283 w308 w330 w350 w386]
      tunnel: ["Bouncer Parameters" w111 w143 w169 w187 w241 w282 w305 w329 w349 w385] -> w28
      tunnel: w27 -> [_ w111 w143 w169 w187 w241 w282 w305 w329 w349 w385]
      frame "Initialize" {
        w70 = 10171 items=["Rising"=10280, "Falling"=10171] ("edge")
        w86 = 10280 items=["Rising"=10280, "Falling"=10171] ("edge")
        w89 = 10123 items=["Finite Samples"=10178, "Continuous Samples"=10123] ("sample mode")
        w92 = 10123 items=["Finite Samples"=10178, "Continuous Samples"=10123, "Hardware Timed Single Point"=12522] ("sample mode")
        w97 = 10214 items=["High"=10192, "Low"=10214] ("idle state")
        w96 = 10364 items=["Seconds"=10364] ("units")
        (unwired) 10000.0 ("rate")
        w105 = 10178 items=["Finite Samples"=10178, "Continuous Samples"=10123] ("sample mode")
        # "Bouncer"
        # "Detector Gate"
        # "Analog Counter"
        # "FC Cups"
        # "Change config file to enable gating"
        # "Prepare Bouncer and Gate"
        # "Prepare SRS and Pixie"
        n8 = call "PixieDownloadBoot.vi"("error in (no error)"=w104) -> ("error out"=w66:errorcluster)  [unwired: 5 in, 5 out]
        n9 = call "CalcBouncerGateLEStates.vi"("Bouncer Settings"="Bouncer Parameters", "SampClk.Rate"="SampClk.Rate") -> ("Bouncer Waveform"=w75:waveform(dbl), "High time"=w90:dbl, "low time"=w91:dbl)  [unwired: 7 in]
        "Bouncer Waveform" <- w75
        n10 = call-poly <vilib>:"DAQmx Create Virtual Channel.vi"("counter"=tag "PXI1Slot4/ctr0" ("Counter(s)"), "error in"=w66) -> ("task out"=w100:refnum<k21>, "error out"=w99:errorcluster)  [unwired: 5 in, 7 out]
        n11 = call-poly <vilib>:"DAQmx Create Virtual Channel.vi"("physical channels"=tag "PXI1Slot4/ao0", "error in"=w66) -> ("task out"=w80:refnum<k21>, "error out"=w81:errorcluster)  [unwired: 7 in, 5 out]
        n12 = property class="DAQmx Timing"(reference=w80, error in=w81, "SampClk.Rate"="SampClk.Rate") -> (reference out=w79:refnum<k21>, error out=w78:errorcluster)
        n13 = call-poly <vilib>:"DAQmx Create Virtual Channel.vi"("high time"=w90, "low time"=w91, "counter"=tag "PXI1Slot4/ctr1", "units"=w96, "error in"=w66, "idle state"=w97, "initial delay"=1e-05) -> ("task out"=w93:refnum<k21>, "error out"=w94:errorcluster)  [unwired: 2 in, 5 out]
        n14 = call-poly <vilib>:"DAQmx Create Virtual Channel.vi"("maximum value"=1.0, "minimum value"=-1.0, "physical channels"=tag "PXI1Slot4/ai0:4", "error in"=w99) -> ("task out"=w74:refnum<k21>, "error out"=w72:errorcluster)  [unwired: 5 in, 5 out]
        n15 = call-poly <vilib>:"DAQmx Timing.vi"("task/channels in"=w79, "sample mode"=w89, "waveform"=w75, "error in"=w78) -> ("task out"=w88:refnum<k21>, "error out"=w87:errorcluster)  [unwired: 10 out]
        n16 = call-poly <vilib>:"DAQmx Timing.vi"("task/channels in"=w93, "sample mode"=w92, "error in"=w94) -> ("task out"=w57:refnum<k21>, "error out"=w55:errorcluster)  [unwired: 1 in, 10 out]
        n17 = call <vilib>:"DAQmx Start Task.vi"("task/channels in"=w57, "error in"=w55) -> ("task out"=w56:refnum<k21>, "error out"=w54:errorcluster)  [unwired: 12 in]
        n18 = call-poly <vilib>:"DAQmx Trigger.vi"("task/channels in"=w74, "source"=tag "/PXI1Slot4/PFI13", "edge"=w70, "error in"=w72) -> ("task out"=w73:refnum<k21>, "error out"=w71:errorcluster)  [unwired: 10 in]
        n19 = call-poly <vilib>:"DAQmx Trigger.vi"("task/channels in"=w88, "source"=tag "/PXI1Slot4/PFI13", "edge"=w86, "error in"=w87) -> ("task out"=w83:refnum<k21>, "error out"=w82:errorcluster)  [unwired: 10 out]
        n20 = call-poly <vilib>:"DAQmx Timing.vi"("task/channels in"=w73, "sample mode"=w105, "samples per channel"="samples per channel", "rate"="SampClk.Rate", "error in"=w71) -> ("task out"=w64:refnum<k21>, "error out"=w63:errorcluster)  [unwired: 2 in, 7 out]
        n21 = property class="DAQmx Channel"(reference=w83, error in=w82, "AO.UseOnlyOnBrdMem"=TRUE) -> (reference out=w61:refnum<k21>, error out=w59:errorcluster)
        n22 = call <vilib>:"DAQmx Start Task.vi"("task/channels in"=w61, "error in"=w59) -> ("task out"=w60:refnum<k21>, "error out"=w58:errorcluster)  [unwired: 12 in]
        n23 = call-poly <vilib>:"DAQmx Write.vi"("task/channels in"=w60, "data"=w75, "error in"=w58) -> ("task out"=w76:refnum<k21>, "error out"=w68:errorcluster)  [unwired: 1 in, 10 out]
        n24 = Merge Errors(w63, w54, w68) -> (w67:errorcluster)
      }
      frame "Idle", Default {
        n25 = Flush Queue(queue=w127, error in (no error)=w124) -> (queue out=w120:refnum<queue>, error out=w118:errorcluster)  [unwired: 1 out]
        n26 = case shown="False" "Stop" {
          tunnel: w120 -> [w134 w139]
          tunnel: [w134 w138] -> w119
          tunnel: w118 -> [w133 w137]
          tunnel: [w133 w136] -> w117
          frame False {
          }
          frame True {
            n27 = Enqueue Element(queue=w139, element=PixieKeithleyDAQstates."Stop", error in (no error)=w137) -> (queue out=w138:refnum<queue>, error out=w136:errorcluster)  [unwired: 2 out]
          }
        }
        n28 = case shown="False" "StartDAQ" {
          tunnel: [PixieKeithleyDAQstates."Idle" ("element") PixieKeithleyDAQstates."Start Run" ("element")] -> w125
          frame False {
            n29 = Wait (ms)(milliseconds to wait=u32 10) -> ()  [unwired: 1 out]
          }
          frame True {
          }
        }
        n30 = Enqueue Element(queue=w119, element=w125, error in (no error)=w117) -> (error out=w122:errorcluster)  [unwired: 3 out]
        n31 = case shown="\"Tuning\"" "Mode" {
          frame "Tuning" {
            n32 = property on="Run Parameters" class="Clust (strict)"("Value"=T5 {"Block time (s)"=0.2, "Max Runtime (s)"=100000.0, "Max Counts"=100000, "C12 Limit"=-1.0, "Max BadBlocks"=100} ("Run Parameters")) -> ()  [unwired: 2 in, 2 out]
          }
          frame "Manual" {
          }
          frame "Run", Default {
            n33 = property on="Run Parameters" class="Clust (strict)"("Value"=T5 {"Block time (s)"=1.0, "Max Runtime (s)"=10.0, "Max Counts"=100000, "C12 Limit"=-1.0, "Max BadBlocks"=0} ("Run Parameters")) -> ()  [unwired: 2 in, 2 out]
          }
        }
      }
      frame "Start Run" {
        w153 = T4[] [enum."Wait", enum."Get Block", enum."Check Data"] items=["Initialize", "Restart Bouncer", "Idle", "Load Wheel", "Load Sample", "Start Run", "Wait", "Get Block", "Check Data", "Check Run", "Check Sample", "Analyse and Display", "Stop DAQ", "Log Data", "Stop"]
        w157 = TRUE
        # "Start Bouncer and Gate\nTrigger DAQ and PIXIE"
        # "Start counter"
        # "Code to trigger sync start goes here"
        # "Start/trigger PIXIE"
        # "Start FC DAQ"
        n34 = Not(x=w157) -> (.not. x?=w158:bool)
        n35 = shared-variable "My Computer\\NOSAMSPixieDAQVars.lvlib\\StartDAQ"(w158, error in=w144) -> (error out=w149:errorcluster)
        n36 = call "PixieStartACQ.vi"("error in (no error)"=w149) -> ("error out"=w162:errorcluster)  [unwired: 2 in, 8 out]
        n37 = call <vilib>:"DAQmx Start Task.vi"("task/channels in"=w151, "error in"=w149) -> ("task out"=w150:refnum<k21>, "error out"=w148:errorcluster)  [unwired: 12 out]
        n38 = call "ElapsedTime.vi"("error in (no error)"=w149, "Mode (Update)"=enum16{"Update", "Init"}."Init") -> ("error out"=w161:errorcluster)  [unwired: 9 out]
        n39 = Merge Errors(w161, w162, w148) -> (w156:errorcluster)
        n40 = for {
          tunnel: w159 -> [w168]
          tunnel: w156 -> [w167]
          tunnel: [w166] -> w155
          tunnel: w153 -> [w165] mode=indexing
          n41 = Enqueue Element(queue=w168, element=w165, error in (no error)=w167) -> (error out=w166:errorcluster)  [unwired: 3 out]
        }
        "Acquiring" <- w157
      }
      frame "Wait" {
        # "Start Cups"
        # "Wait for pixie and SRS to get one block of data"
        n42 = call <vilib>:"DAQmx Start Task.vi"("task/channels in"=w171, "error in"=w173) -> ("task out"=w170:refnum<k21>, "error out"=w174:errorcluster)  [unwired: 12 out]
        n43 = Unbundle By Name(w179) -> ("Block time (s)"=w181:dbl)
        n44 = Multiply(x=w181, y=1000.0) -> (x*y=w180:dbl)
        n45 = flat-sequence {
          tunnel: w180 -> [w186]
          tunnel: w174 -> [w185]
          tunnel: [w185] -> w172
          frame #0 {
            n46 = Wait (ms)(milliseconds to wait=w186) -> ()  [unwired: 1 out]
          }
        }
      }
      frame "Get Block" {
        # "Stop cups"
        # "LT&RT won't be accurate unless PIXIE is stopped."
        # "Problem: PIXIE & FCs not synched."
        n47 = call-poly <vilib>:"DAQmx Read.vi"("task/channels in"=w240, "number of samples per channel"=-1, "timeout"=10.0, "error in"=w215) -> ("task out"=w191:refnum<k21>, "data"=w223:waveform(dbl)[], "error out"=w189:errorcluster)  [unwired: 9 out]
        n48 = call "ProcessFCCurrentsLE.vi"("FC Data"=w223, "Bouncer Settings"=w187, "FC Offset"="FC Offset") -> ("Mean Currents"=w221:dbl[], "Output Waveforms"=w222:waveform(dbl)[])  [unwired: 7 in]
        n49 = Index Array(array=w222) -> (element #1=→"HE 12C Cup":waveform(dbl), element #2=→"LE 12C Cup":waveform(dbl), element #3=→"HE 13CH Cup":waveform(dbl), element #4=→"HE 13CL Cup":waveform(dbl), element #5=→"LE 13C Cup":waveform(dbl), element #6=→"Bouncer":waveform(dbl))  [unwired: 6 in]
        n50 = call <vilib>:"DAQmx Stop Task.vi"("task/channels in"=w191, "error in"=w189) -> ("task out"=w190:refnum<k21>, "error out"=w188:errorcluster)  [unwired: 12 out]
        n51 = call "PixieGetData.vi"("error IO"=w188) -> ("error out"=w214:errorcluster, "PixieTimes"=w224:T9, "Histogram Data"=w203:u32[][], 3:w231, 4:w204, 5:w234, 6:→"CH0 SFDT", 7:w205, 11:→"CH0 GDT")  [unwired: 2 in]
        "Block Spectrum" <- w234
        "Ch0 LT" <- w231
        "Ch1 LT" <- w203
        "Run time [s]" <- w224
        "CH1 SFDT" <- w204
        "CH1 GDT" <- w205
        n52 = Index Array(array=w221) -> (element #1=w210:dbl, element #2=w199:dbl, element #3=w209:dbl, element #4=w208:dbl, element #5=w198:dbl)  [unwired: 5 in]
        "C13H" <- w209
        "C13L" <- w208
        "C12" <- w210
        "C12LE" <- w199
        "C13LE" <- w198
        n53 = property on="Block Spectrum" class="WFGraph (strict)"() -> ("CrsrList"=w233:T10)  [unwired: 2 in, 2 out]
        n54 = call "PixieCalcCountData.vi"("CrsrList"=w233, "Histogram Data"=w234, "CH0 LT"=w231, "CH1 LT"=w203) -> ("Count Data"=w232:T11)  [unwired: 1 in]
        n55 = Add(x=w209, y=w208) -> (x+y=w219:dbl)
        n56 = Divide(x=w209, y=w208) -> (x/y=→"13C H/L":dbl)
        n57 = Unbundle By Name(w232) -> ("Ch0 Counts"=→"Ch0 Counts":u32, "Ch0 Rate"=→"Ch0 Rate":dbl, "Ch1 Counts"=w202:u32, "Ch1 Rate"=→"Ch1 Rate":dbl)
        "Ch1 Counts" <- w202
        n58 = Bundle(w210, w219) -> (→"Currents":cluster{dbl, dbl})  [unwired: 1 out]
        n59 = Add(x=w204, y=w205) -> (x+y=w206:dbl)
        n60 = Subtract(x=w203, y=w206) -> (x-y=w201:dbl[][])
        n61 = call "InsertBlockData.vi"("C12LE"=w199, "C12"=w210, "Block Data In"=w216, "C13H"=w209, "C13L"=w208, "C13LE"=w198, "Counts"=w202, "LT"=w201, "RT"=w224) -> ("Block Data Out"=w235:T8)  [unwired: 6 in]
        n62 = Divide(x=w202, y=w201) -> (x/y=w200:dbl[][])
        "DT Corrected Rate" <- w200
        n63 = Bundle(w210, w219, w200, w199, w198) -> (→"Currents & Counts":cluster{dbl, dbl, dbl[][], dbl, dbl})  [unwired: 1 out]
      }
      frame "Check Data" {
        # "check if stats reqs satisfied\nwrite to logfile"
        # "Check block data"
        # "Check data quality\n    add to run data if good\n    discard, increment bad block counter\n     get new block if bad"
        n64 = Unbundle By Name(w253) -> ("C12"=w256:dbl[])
        n65 = Unbundle By Name(w249) -> ("C12 Limit"=w258:dbl, "Max BadBlocks"=w252:u8)
        n66 = case shown="False" "Stop DAQ" {
          tunnel: w251 -> [w260 w263]
          tunnel: [w260 w262] -> w250
          frame False {
          }
          frame True {
            n67 = Enqueue Element(queue=w263, element=PixieKeithleyDAQstates."Stop DAQ" ("Next State")) -> (queue out=w262:refnum<queue>)  [unwired: 1 in, 3 out]
          }
        }
        n68 = Delete From Array(array=w256) -> (deleted portion=w255:dbl)  [unwired: 2 in, 1 out]
        n69 = Greater?(x=w255, y=w258) -> (0:w254:bool)
        "Good Block" <- w254
        n70 = case shown="True" w254 {
          tunnel: [w273 w277] -> w243
          tunnel: w242 -> [w274 w278]
          tunnel: w253 -> [_ w279]
          tunnel: w252 -> [w272 _]
          tunnel: w250 -> [w270 w281]
          frame False {
            w267 = T4[] [enum."Wait", enum."Get Block", enum."Check Data"] items=["Initialize", "Restart Bouncer", "Idle", "Load Wheel", "Load Sample", "Start Run", "Wait", "Get Block", "Check Data", "Check Run", "Check Sample", "Analyse and Display", "Stop DAQ", "Log Data", "Stop"]
            w269 = T4[] [enum."Stop DAQ"] items=["Initialize", "Restart Bouncer", "Idle", "Load Wheel", "Load Sample", "Start Run", "Wait", "Get Block", "Check Data", "Check Run", "Check Sample", "Analyse and Display", "Stop DAQ", "Log Data", "Stop"]
            # "Bad Block"
            n71 = Unbundle By Name(w274) -> ("BadBlocks"=w266:u8)
            n72 = Decrement(x=w272) -> (x-1=w265:u8)
            n73 = Increment(x=w266) -> (x+1=w264:u8)
            n74 = Bundle By Name(cluster=w274, "BadBlocks"=w264) -> (w273:T3)
            n75 = Greater Or Equal?(x=w264, y=w265) -> (x >= y?=w271:bool)
            n76 = Select(t=w269, s=w271, f=w267) -> (s? t:f=w268:T4[])
            n77 = for {
              tunnel: w268 -> [w276] mode=indexing
              tunnel: w270 -> [w275]
              n78 = Enqueue Element(queue=w275, element=w276) -> ()  [unwired: 1 in, 4 out]
            }
          }
          frame True {
            n79 = call "PKDAQAppendBlockDataCont.vi"("Run Summary"=w278, "Block Data"=w279) -> ("Run Summary Out"=w277:T3)  [unwired: 9 out]
            n80 = Enqueue Element(queue=w281, element=PixieKeithleyDAQstates."Check Run") -> ()  [unwired: 1 in, 4 out]
          }
        }
        "Summary Data" <- w243
      }
      frame "Check Run" {
        # "Get another block?"
        n81 = Unbundle By Name(w289) -> ("Max Counts"=w299:u32, "Max Runtime (s)"=w298:dbl)
        n82 = Unbundle By Name(w293) -> ("Counts"=w295:u32, "LT"=w294:dbl)
        n83 = Less?(x=w299, y=w295) -> (x < y?=w291:bool)
        n84 = Greater Or Equal?(x=w294, y=w298) -> (x >= y?=w290:bool)
        n85 = Or(x=w291, y=w290) -> (x .or. y?=w292:bool)
        n86 = case shown="True" w292 {
          tunnel: [w303 w304] -> w288
          frame False {
            w303 = T4[] [enum."Analyse and Display", enum."Wait", enum."Get Block", enum."Check Data"] items=["Initialize", "Restart Bouncer", "Idle", "Load Wheel", "Load Sample", "Start Run", "Wait", "Get Block", "Check Data", "Check Run", "Check Sample", "Analyse and Display", "Stop DAQ", "Log Data", "Stop"]
          }
          frame True {
            w304 = T4[] [enum."Analyse and Display", enum."Stop DAQ"] items=["Initialize", "Restart Bouncer", "Idle", "Load Wheel", "Load Sample", "Start Run", "Wait", "Get Block", "Check Data", "Check Run", "Check Sample", "Analyse and Display", "Stop DAQ", "Log Data", "Stop"]
          }
        }
        n87 = for {
          tunnel: w287 -> [w302]
          tunnel: w288 -> [w301] mode=indexing
          n88 = Enqueue Element(queue=w302, element=w301) -> ()  [unwired: 1 in, 4 out]
        }
      }
      frame "Analyse and Display" {
        n89 = call "PKDAQRunningAvg.vi"("Block Data"=w306, "CountPoints"="CountPoints", "CurPoints"="CurPoints") -> ("RunningAverages"=w324:T3)  [unwired: 8 out]
        "RunningAverages" <- w324
        n90 = call "CalcRatiosBouncer.vi"("Run Summary"=w324) -> ("Run Ratios"=w320:T7)  [unwired: 10 out]
        "Moving Averages" <- w320
        n91 = call "CalcRatiosBouncer.vi"("Run Summary"=w307) -> ("Run Ratios"=w311:T7)  [unwired: 10 out]
        "Run Average Ratios" <- w311
        n92 = Unbundle By Name(w311) -> ("C14Rate"=w323:dbl)
        n93 = Unbundle By Name(w320) -> ("C14Rate"=w321:dbl)
        n94 = Unbundle By Name(w311) -> ("C14/12"=w319:dbl, "d13C"=w314:dbl)
        n95 = Unbundle By Name(w320) -> ("C14/12"=w318:dbl, "d13C"=w313:dbl, "C13/12"=w317:dbl)
        n96 = Reciprocal(x=w317) -> (1/x=→"12/13":dbl)
        n97 = Bundle("C14Rate"=w323, "C14Rate"=w321) -> (→"Ch1 Rate 2":cluster{"C14Rate":dbl, "C14Rate":dbl})  [unwired: 1 out]
        n98 = Bundle("C14/12"=w319, "C14/12"=w318, "d13C"=w314, "d13C"=w313) -> (→"Ratios":T6)  [unwired: 1 out]
      }
      frame "Stop DAQ" {
        n99 = call "PixieStopACQ.vi"("error in (no error)"=w336) -> ("error out"=w340:errorcluster)  [unwired: 10 out]
        n100 = call "PixieCheckRunStatus.vi"("error in (no error)"=w340) -> ("error out"=w334:errorcluster, "run finished"=w339:bool)  [unwired: 1 in, 8 out]
        n101 = case shown="True" w339 {
          tunnel: w338 -> [w344 w346]
          frame False {
            n102 = Enqueue Element(queue=w344, element=PixieKeithleyDAQstates."Stop DAQ" ("Next State")) -> ()  [unwired: 1 in, 4 out]
          }
          frame True {
            w345 = T4[] [enum."Get Block", enum."Check Data", enum."Analyse and Display", enum."Log Data", enum."Idle"] items=["Initialize", "Restart Bouncer", "Idle", "Load Wheel", "Load Sample", "Start Run", "Wait", "Get Block", "Check Data", "Check Run", "Check Sample", "Analyse and Display", "Stop DAQ", "Log Data", "Stop"]
            n103 = for {
              tunnel: w346 -> [w348]
              tunnel: w345 -> [w347] mode=indexing
              n104 = Enqueue Element(queue=w348, element=w347) -> ()  [unwired: 1 in, 4 out]
            }
          }
        }
      }
      frame "Log Data" {
        # "Add data to status file and return here?"
        # "Return to DAQ Control\nData if good run\nError condition if bad"
        n105 = call "ElapsedTime.vi"("error in (no error)"=w360) -> ("error out"=w359:errorcluster, "Elapsed Time"=w358:dbl)  [unwired: 1 in, 8 out]
        "Elapsed Time" <- w358
        n106 = call-poly <vilib>:"DAQmx Read.vi"("task/channels in"=w364, "error in"=w359) -> ("task out"=w363:refnum<k21>, "data"=w357:u32, "error out"=w362:errorcluster)  [unwired: 1 in, 10 out]
        "SCA Counts" <- w357
        n107 = call <vilib>:"DAQmx Stop Task.vi"("task/channels in"=w363, "error in"=w362) -> ("task out"=w361:refnum<k21>, "error out"=w353:errorcluster)  [unwired: 12 out]
        n108 = Unbundle By Name(w370) -> ("d13C"=w369:dbl, "C14/12"=w368:dbl)
        n109 = Unbundle By Name(w355) -> ("C12"=w383:dbl, "C13L"=w367:dbl, "C13H"=w365:dbl, "Counts"=w382:u32, "LT"=w381:dbl, "RT"=w380:dbl)
        n110 = shared-variable "My Computer\\NOSAMSPixieDAQVars.lvlib\\C13HCur"(w365) -> ()  [unwired: 2 out]
        n111 = shared-variable "My Computer\\NOSAMSPixieDAQVars.lvlib\\C12Cur"(w383) -> ()  [unwired: 2 out]
        n112 = shared-variable "My Computer\\NOSAMSPixieDAQVars.lvlib\\C13LCur"(w367) -> ()  [unwired: 2 out]
        n113 = shared-variable "My Computer\\NOSAMSPixieDAQVars.lvlib\\Runtime"(w380) -> ()  [unwired: 2 out]
        n114 = shared-variable "My Computer\\NOSAMSPixieDAQVars.lvlib\\Livetime"(w381) -> ()  [unwired: 2 out]
        n115 = shared-variable "My Computer\\NOSAMSPixieDAQVars.lvlib\\Counts"(w382) -> ()  [unwired: 2 out]
        n116 = shared-variable "My Computer\\NOSAMSPixieDAQVars.lvlib\\d13C"(w369) -> ()  [unwired: 1 in, 1 out]
        n117 = shared-variable "My Computer\\NOSAMSPixieDAQVars.lvlib\\C1412"(w368) -> ()  [unwired: 1 in, 1 out]
        n118 = Add(x=w367, y=w365) -> (x+y=w366:dbl)
        n119 = Divide(x=w357, y=w358) -> (x/y=→"SCA Rate":dbl)
        n120 = shared-variable "My Computer\\NOSAMSPixieDAQVars.lvlib\\C13"(w366) -> ()  [unwired: 1 in, 1 out]
        n121 = Build Path(base path="Log File Path", name or relative path="Logfile") -> (appended path=w374:path)
        n122 = call "CreateLogfile.vi"("error in (no error)"=w353, "Log File Path"=w374) -> ("error out"=w384:errorcluster)  [unwired: 1 in, 8 out]
        n123 = call "BouncerDAQinit.vi"("error in (no error)"=w384) -> ("error out"=w351:errorcluster, "Run Ratios"=w373:T7, "Summary Data"=w372:T3, "Block Data"=w371:T8)  [unwired: 1 in, 6 out]
        n124 = shared-variable "My Computer\\NOSAMSPixieDAQVars.lvlib\\Acquiring"(FALSE ("Acquire"), error in=w351) -> (error out=w377:errorcluster)
      }
      frame "Stop" {
        n125 = Enqueue Element(queue=w393, element=PixieKeithleyDAQstates."Stop" ("Next State")) -> ()  [unwired: 1 in, 4 out]
      }
    }
    n126 = Equal?(x=w37, y=PixieKeithleyDAQstates."Stop" ("States")) -> (x = y?=w52:bool)
  }
  n127 = call <vilib>:"DAQmx Clear Task.vi"("task in"=w4, "error in"=w2) -> ("error out"=w3:errorcluster)  [unwired: 13 out]
  n128 = call <vilib>:"DAQmx Clear Task.vi"("task in"=w5, "error in"=w3) -> ("error out"=w1:errorcluster)  [unwired: 13 out]
  n129 = call <vilib>:"DAQmx Clear Task.vi"("task in"=w26, "error in"=w1) -> ("error out"=w8:errorcluster)  [unwired: 13 out]
  n130 = call <vilib>:"DAQmx Clear Task.vi"("task in"=w6, "error in"=w8) -> ("error out"=w7:errorcluster)  [unwired: 13 out]
  n131 = Release Queue(queue=w20, error in (no error)=w7) -> (error out=w13:errorcluster)  [unwired: 3 out]
  n132 = call <vilib>:"General Error Handler.vi"("error in (no error)"=w13) -> ("error out"=→"error out":errorcluster)  [unwired: 1 in, 13 out]
